vi "get-nodes.vi"(8 "error in (no error)":errorcluster, 11 "Graph in":refnum<class "Graph.lvclass">) -> (0 "error out":errorcluster, 2 "nodes":refnum<class "Node.lvclass">[](array[class]), 3 "Graph out":refnum<class "Graph.lvclass">)   [LabVIEW 2020, in "graph.lvlib" / "Graph.lvclass"]
uses:
  Graph.lvclass
  Node/Node.lvclass
  Graph.lvclass/Graph.ctl
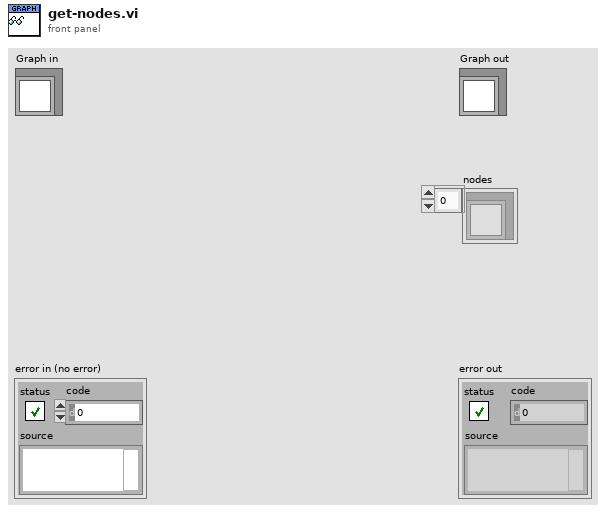
[diagram p1: front panel]
types:
  T1 = map{refnum<class "ID.lvclass">, refnum<class "Node.lvclass">}
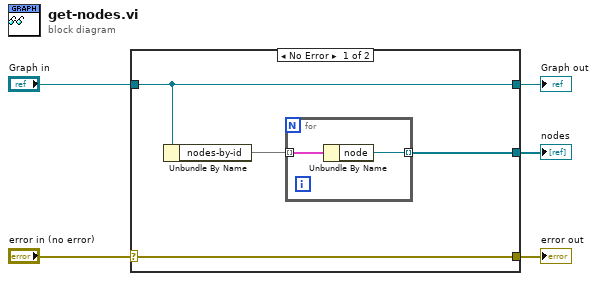
[diagram p0: block diagram]
diagram:
  n1 = case shown="No Error" "error in (no error)" {
    selector: "error in (no error)" -> [w9 w12]
    tunnel: [w9 w12] -> w4
    tunnel: [w8 w13] -> w2
    tunnel: "Graph in" -> [w8 w13]
    tunnel: [w6 _] -> w1
    frame No Error {
      n2 = Unbundle By Name(w8) -> ("nodes-by-id"=w7:T1)
      n3 = for {
        tunnel: w7 -> [w11] mode=indexing
        tunnel: [w10] -> w6 mode=indexing
        n4 = Unbundle By Name(w11) -> ("node"=w10:refnum<class "Node.lvclass">)
      }
    }
    frame Error {
    }
  }
  "error out" <- w4
  "Graph out" <- w2
  "nodes" <- w1
